vi "find alias from UID.vi"(10 "UID":string, 11 "instance data":T1[](array[typedef])) -> (3 "Alias":string)   [LabVIEW 2025, in "CEF.lvlib"]
doc: "Searches a set of flattened instances for a given ID and returns the alias associated with that ID.Copyright 2017 National Instruments Corporation\n\nLicensed under the Apache License, Version 2.0 (the \"License\"); you may not use this file except in compliance with the License. You may obtain a copy of the License at http://www.apache.org/licenses/LICENSE-2.0\nUnless required by applicable law or agreed to in writing, software distributed under the License is distributed on an \"AS IS\" BASIS, WITHOUT WARRANTIES OR CONDITIONS OF ANY KIND, either express or implied. See the License for the specific language governing permissions and limitations under the License."
uses:
  CEF.lvlib
  instance data.ctl
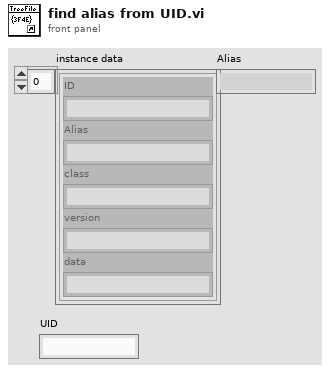
[diagram p1: front panel]
types:
  T1 = typedef "CEF.lvlib/instance data.ctl" = cluster{"ID":string, "Alias":string, "class":string, "version":string, "data":string}
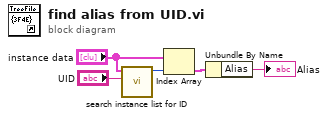
[diagram p0: block diagram]
diagram:
  n1 = call "search instance list for ID.vi"("UID"="UID", "instance data"="instance data") -> ("index"=w3:i32)  [unwired: 9 in]
  n2 = Index Array(array="instance data", index=w3) -> (element=w2:T1)
  n3 = Unbundle By Name(w2) -> ("Alias"=→"Alias":string)
